vi "create_datetime_folder.vi"(8 "error in (no error)":errorcluster, 11 "Path":path) -> (0 "error out":errorcluster, 3 "created path":path)   [LabVIEW 2011, in "Fiberscope_library.lvlib"]
uses:
  Fiberscope_library.lvlib
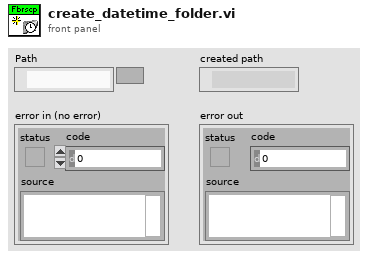
[diagram p1: front panel]
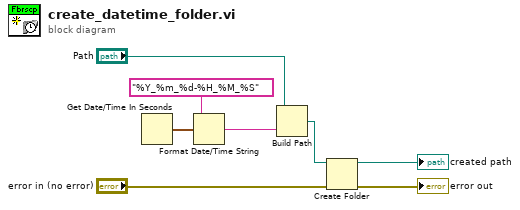
[diagram p0: block diagram]
diagram:
  n1 = Get Date/Time In Seconds() -> (seconds since 1Jan1904=w2:timestamp)
  n2 = Format Date/Time String(time format string (%c)="%Y_%m_%d-%H_%M_%S", seconds (now)=w2) -> (date/time string=w3:string)  [unwired: 1 in]
  n3 = Build Path(base path="Path", name or relative path=w3) -> (appended path=w5:path)
  n4 = Create Folder(path (use dialog)=w5, error in="error in (no error)") -> (created path=→"created path":path, error out=→"error out":errorcluster)  [unwired: 1 in, 1 out]
